vi "Draw Delta Values line.vi"(8 "error in (no error)":errorcluster, 9 "Coords-end":T2, 10 "Coords-start":T2, 11 "PlotAreaBounds":T1) -> (0 "error out":errorcluster, 3 "picture":picture)   [LabVIEW 2021, in "RocketPlot.lvlib"]
uses:
  RocketPlot.lvlib
  <vilib>/Utility/miscctls.llb/LVPoint32TypeDef.ctl
  <vilib>/Utility/miscctls.llb/LVRectTypeDef.ctl
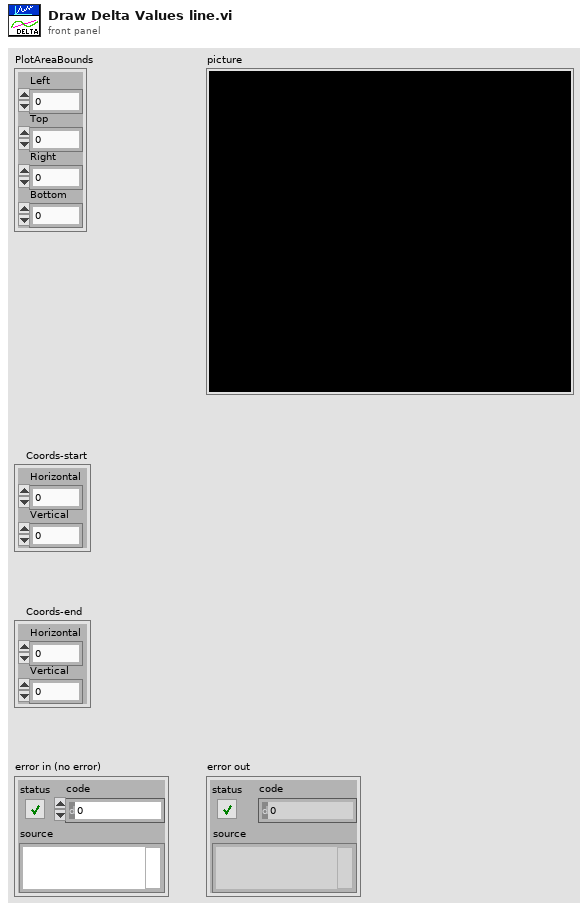
[diagram p1: front panel]
types:
  T1 = typedef "LVRectTypeDef.ctl" = cluster{"Left":i16, "Top":i16, "Right":i16, "Bottom":i16}
  T2 = typedef "LVPoint32TypeDef.ctl" = cluster{"Horizontal":i32, "Vertical":i32}
  T3 = cluster{"Width":u16, "Style":enum32{"Solid", "Dash", "Dot", "DashDot", "DashDotDot"}}
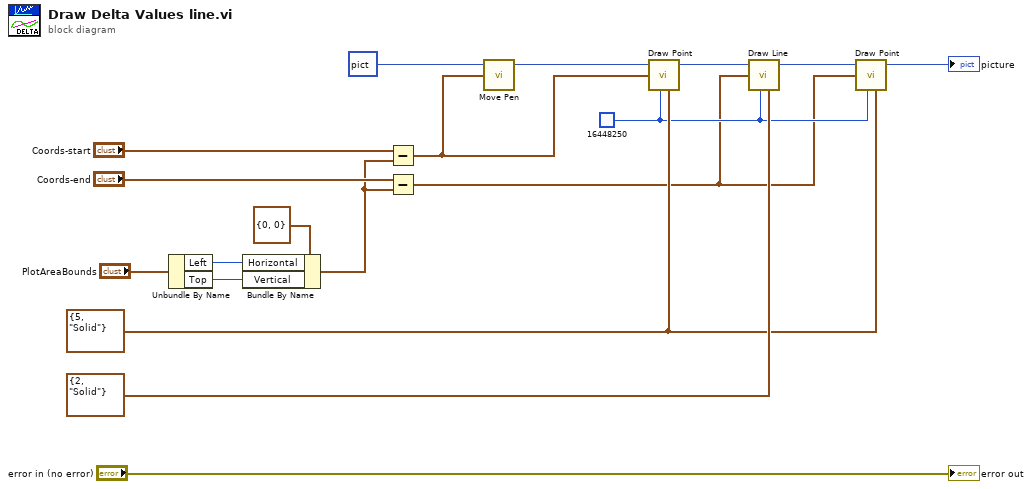
[diagram p0: block diagram]
diagram:
  w10 = u32 16448250 ("color(black)")
  w11 = T3 {"Width"=5, "Style"=enum."Solid"} ("pen")
  n1 = Unbundle By Name("PlotAreaBounds") -> ("Left"=w4:i16, "Top"=w3:i16)
  n2 = Bundle By Name(cluster=T2 {"Horizontal"=0, "Vertical"=0} ("Coords"), "Horizontal"=w4, "Vertical"=w3) -> (w1:T2)
  n3 = Subtract(x="Coords-start", y=w1) -> (x-y=w8:T2)
  n4 = Subtract(x="Coords-end", y=w1) -> (x-y=w6:T2)
  n5 = call <vilib>:"Move Pen.vi"("new position"=w8, "picture"=picture data[5B]) -> ("new picture"=w15:picture)  [unwired: 3 in]
  n6 = call <vilib>:"Draw Point.vi"("picture"=w15, "point(x,y)"=w8, "color(black)"=w10, "pen"=w11) -> ("new picture"=w14:picture)  [unwired: 5 in]
  n7 = call <vilib>:"Draw Line.vi"("picture"=w14, "end point"=w6, "color(black)"=w10, "pen"=T3 {"Width"=2, "Style"=enum."Solid"}) -> ("new picture"=w13:picture)  [unwired: 5 in]
  n8 = call <vilib>:"Draw Point.vi"("picture"=w13, "point(x,y)"=w6, "color(black)"=w10, "pen"=w11) -> ("new picture"=→"picture":picture)  [unwired: 5 in]
  "error out" <- "error in (no error)"
